vi "Instrument Info To Log.vi"(0 "Instrument Info":T1, 11 "error in (no error)":errorcluster) -> (15 "error out":errorcluster)   [LabVIEW 2018]
uses:
  Station/Station Support/Controls/Instrument Info.ctl
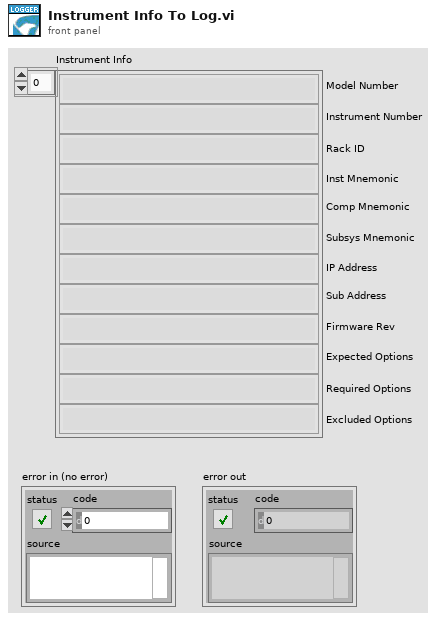
[diagram p1: front panel]
types:
  T1 = typedef "Instrument Info.ctl" = string[]
  T2 = cluster{"Log File Input":string, "Log Entry Type":enum16{"STANDARD", "WARNING", "CRITICAL"}}
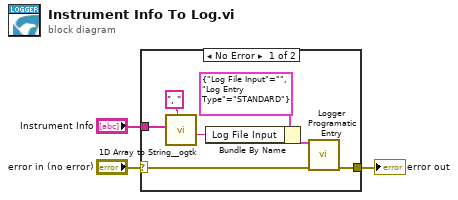
[diagram p0: block diagram]
diagram:
  n1 = case shown="No Error" "error in (no error)" {
    selector: "error in (no error)" -> [w5 w11]
    tunnel: [w4 w11] -> w2
    tunnel: "Instrument Info" -> [w6 _]
    frame No Error {
      n2 = call <userlib>:"1D Array to String__ogtk.vi"("delimiter (Tab)"=", ", "Array of Strings"=w6) -> ("delimited string"=w8:string)  [unwired: 9 in]
      n3 = Bundle By Name(cluster=T2 {"Log File Input"="", "Log Entry Type"=enum."STANDARD"} ("Log File Input"), "Log File Input"=w8) -> (w10:T2)
      n4 = call "Logger Programatic Entry.vi"("Log File Input"=w10, "error in (no error)"=w5) -> ("error out"=w4:errorcluster)  [unwired: 13 in]
    }
    frame Error {
    }
  }
  "error out" <- w2
